vi "Close.vi"(8 "error in (no error)":errorcluster, 11 "AutoComplete in":refnum<class "AutoComplete.lvclass">) -> (0 "error out":errorcluster)   [LabVIEW 2020, in "AutoComplete.lvlib" / "AutoComplete.lvclass"]
doc: "Closes the autocomplete handler. Autocomplete behavior will stop once this VI is called."
uses:
  AutoComplete.lvclass
  AutoComplete.lvclass/AutoComplete.ctl
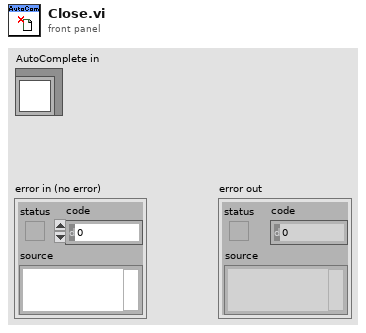
[diagram p1: front panel]
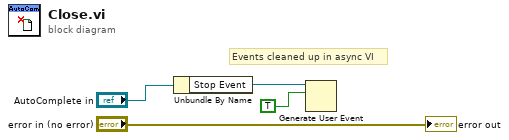
[diagram p0: block diagram]
diagram:
  # "Events cleaned up in async VI"
  n1 = Unbundle By Name("AutoComplete in") -> ("Stop Event"=w2:refnum<user-event>)
  n2 = Generate User Event(user event=w2, event data cluster=TRUE ("event data")) -> ()  [unwired: 2 in, 2 out]
  "error out" <- "error in (no error)"
